vi "HFRR ADV v03.vi"() -> ()   [LabVIEW 2025] (continued)
            n1403 = Delete From Array(array=w1051, index=0) -> (array with subset deleted=w926:dbl[])  [unwired: 1 in, 1 out]
            n1404 = Delete From Array(array=w1031, index=0) -> (array with subset deleted=w1011:dbl[])  [unwired: 1 in, 1 out]
            n1405 = Delete From Array(array=w1001, index=0) -> (array with subset deleted=w928:dbl[])  [unwired: 1 in, 1 out]
            n1406 = Delete From Array(array=w1039, index=0) -> (array with subset deleted=w1012:dbl[])  [unwired: 1 in, 1 out]
            n1407 = Delete From Array(array=w1049, index=0) -> (array with subset deleted=w1010:dbl[])  [unwired: 1 in, 1 out]
            n1408 = Delete From Array(array=w1058, index=0) -> (array with subset deleted=w1013:dbl[])  [unwired: 1 in, 1 out]
            n1409 = Bundle "Bundle"(w922, w1011) -> (w1076:cluster{dbl[], dbl[]})  [unwired: 1 in]
            n1410 = Bundle "Bundle"(w926, w1010) -> (w1078:cluster{dbl[], dbl[]})  [unwired: 1 in]
            n1411 = Bundle "Bundle"(w924, w1012) -> (w1077:cluster{dbl[], dbl[]})  [unwired: 1 in]
            n1412 = Bundle "Bundle"(w928, w1013) -> (w947:cluster{dbl[], dbl[]})  [unwired: 1 in]
            n1413 = Build Array "Build Array"(w947, w1078, w1077, w1076) -> (→"Coefficient Of Friction":cluster{dbl[], dbl[]}[])
            n1414 = Delete From Array(array=w1046, index=0) -> (array with subset deleted=w1047:dbl[])  [unwired: 1 in, 1 out]
            n1415 = Delete From Array(array=w1028, index=0) -> (array with subset deleted=w1029:dbl[])  [unwired: 1 in, 1 out]
            n1416 = Delete From Array(array=w1037, index=0) -> (array with subset deleted=w1038:dbl[])  [unwired: 1 in, 1 out]
            n1417 = Delete From Array(array=w1055, index=0) -> (array with subset deleted=w1056:dbl[])  [unwired: 1 in, 1 out]
            n1418 = Delete From Array(array=w1026, index=0) -> (array with subset deleted=w956:dbl[])  [unwired: 1 in, 1 out]
            n1419 = Delete From Array(array=w1035, index=0) -> (array with subset deleted=w957:dbl[])  [unwired: 1 in, 1 out]
            n1420 = Delete From Array(array=w1053, index=0) -> (array with subset deleted=w959:dbl[])  [unwired: 1 in, 1 out]
            n1421 = Delete From Array(array=w1044, index=0) -> (array with subset deleted=w958:dbl[])  [unwired: 1 in, 1 out]
            n1422 = Bundle "Bundle"(w922, w956) -> (w1068:cluster{dbl[], dbl[]})  [unwired: 1 in]
            n1423 = Bundle "Bundle"(w926, w958) -> (w1069:cluster{dbl[], dbl[]})  [unwired: 1 in]
            n1424 = Bundle "Bundle"(w924, w957) -> (w1067:cluster{dbl[], dbl[]})  [unwired: 1 in]
            n1425 = Bundle "Bundle"(w928, w959) -> (w946:cluster{dbl[], dbl[]})  [unwired: 1 in]
            n1426 = Delete From Array(array=w1019, index=0) -> (array with subset deleted=w1007:dbl[])  [unwired: 1 in, 1 out]
            n1427 = Build Array "Build Array"(w946, w1069, w1067, w1068) -> (→"Air Temperature":cluster{dbl[], dbl[]}[])
            n1428 = Delete From Array(array=w1024, index=0) -> (array with subset deleted=w1009:dbl[])  [unwired: 1 in, 1 out]
            "array w/ subset deleted" <- w1009
            n1429 = Delete From Array(array=w1022, index=0) -> (array with subset deleted=w1008:dbl[])  [unwired: 1 in, 1 out]
            n1430 = Delete From Array(array=w999, index=0) -> (array with subset deleted=w955:dbl[])  [unwired: 1 in, 1 out]
            n1431 = Bundle "Bundle"(w922, w1029) -> (w1061:cluster{dbl[], dbl[]})  [unwired: 1 in]
            n1432 = Bundle "Bundle"(w926, w1047) -> (w1060:cluster{dbl[], dbl[]})  [unwired: 1 in]
            n1433 = Bundle "Bundle"(w924, w1038) -> (w1062:cluster{dbl[], dbl[]})  [unwired: 1 in]
            n1434 = Bundle "Bundle"(w928, w1056) -> (w920:cluster{dbl[], dbl[]})  [unwired: 1 in]
            n1435 = Build Array "Build Array"(w920, w1060, w1062, w1061) -> (→"XY Graph 13":cluster{dbl[], dbl[]}[])
            n1436 = Delete From Array(array=w1018, index=0) -> (array with subset deleted=w1006:dbl[])  [unwired: 1 in, 1 out]
            n1437 = Delete From Array(array=w993, index=0) -> (array with subset deleted=w952:dbl[])  [unwired: 1 in, 1 out]
            n1438 = Delete From Array(array=w997, index=0) -> (array with subset deleted=w954:dbl[])  [unwired: 1 in, 1 out]
            n1439 = Delete From Array(array=w995, index=0) -> (array with subset deleted=w953:dbl[])  [unwired: 1 in, 1 out]
            n1440 = call-poly <vilib>:"Mean.vi"("X"=w1011) -> ("mean"=→"КОФ4":dbl)  [unwired: 1 out]
            n1441 = call-poly <vilib>:"Mean.vi"("X"=w1013) -> ("mean"=→"КОФ1":dbl)  [unwired: 1 out]
            n1442 = call-poly <vilib>:"Mean.vi"("X"=w1012) -> ("mean"=→"КОФ3":dbl)  [unwired: 1 out]
            n1443 = Bundle "Bundle"(w928, w1009) -> (w942:cluster{dbl[], dbl[]})  [unwired: 1 in]
            n1444 = Bundle "Bundle"(w922, w1006) -> (w1014:cluster{dbl[], dbl[]})  [unwired: 1 in]
            n1445 = Bundle "Bundle"(w926, w1008) -> (w1016:cluster{dbl[], dbl[]})  [unwired: 1 in]
            n1446 = Bundle "Bundle"(w924, w1007) -> (w1015:cluster{dbl[], dbl[]})  [unwired: 1 in]
            n1447 = call-poly <vilib>:"Mean.vi"("X"=w1010) -> ("mean"=→"КОФ2":dbl)  [unwired: 1 out]
            n1448 = Build Array "Build Array"(w942, w1016, w1015, w1014) -> (→"Sample Temperature":cluster{dbl[], dbl[]}[])
            n1449 = Bundle "Bundle"(w928, w955) -> (w919:cluster{dbl[], dbl[]})  [unwired: 1 in]
            n1450 = Bundle "Bundle"(w922, w952) -> (w990:cluster{dbl[], dbl[]})  [unwired: 1 in]
            n1451 = Bundle "Bundle"(w926, w954) -> (w992:cluster{dbl[], dbl[]})  [unwired: 1 in]
            n1452 = Bundle "Bundle"(w924, w953) -> (w991:cluster{dbl[], dbl[]})  [unwired: 1 in]
            n1453 = Delete From Array(array=w978, index=0) -> (array with subset deleted=w950:dbl[])  [unwired: 1 in, 1 out]
            n1454 = Delete From Array(array=w976, index=0) -> (array with subset deleted=w949:dbl[])  [unwired: 1 in, 1 out]
            n1455 = call-poly <vilib>:"Mean.vi"("X"=w1008) -> ("mean"=→"CP2":dbl)  [unwired: 1 out]
            n1456 = call-poly <vilib>:"Mean.vi"("X"=w1006) -> ("mean"=→"CP4":dbl)  [unwired: 1 out]
            n1457 = Build Array "Build Array"(w919, w992, w991, w990) -> (→"Humidity":cluster{dbl[], dbl[]}[])
            n1458 = call-poly <vilib>:"Mean.vi"("X"=w1007) -> ("mean"=→"CP3":dbl)  [unwired: 1 out]
            n1459 = call-poly <vilib>:"Mean.vi"("X"=w1009) -> ("mean"=→"CP1":dbl)  [unwired: 1 out]
            n1460 = Delete From Array(array=w980, index=0) -> (array with subset deleted=w951:dbl[])  [unwired: 1 in, 1 out]
            n1461 = Bundle "Bundle"(w959, w955) -> (w961:cluster{dbl[], dbl[]})  [unwired: 1 in]
            n1462 = Bundle "Bundle"(w956, w952) -> (w964:cluster{dbl[], dbl[]})  [unwired: 1 in]
            n1463 = Bundle "Bundle"(w958, w954) -> (w962:cluster{dbl[], dbl[]})  [unwired: 1 in]
            n1464 = Bundle "Bundle"(w957, w953) -> (w963:cluster{dbl[], dbl[]})  [unwired: 1 in]
            n1465 = Delete From Array(array=w974, index=0) -> (array with subset deleted=w948:dbl[])  [unwired: 1 in, 1 out]
            n1466 = Build Array "Build Array"(w961, w962, w963, w964) -> (→"Air Temp vs Rh":cluster{dbl[], dbl[]}[])
            n1467 = Build Array "Build Array"(w919, w942) -> (w945:cluster{dbl[], dbl[]}[])
            "XY Graph 17" <- w945
            n1468 = local write "XY Graph 16"(w945) -> ()
            n1469 = Bundle "Bundle"(w926, w950) -> (w972:cluster{dbl[], dbl[]})  [unwired: 1 in]
            n1470 = Bundle "Bundle"(w924, w949) -> (w971:cluster{dbl[], dbl[]})  [unwired: 1 in]
            n1471 = Bundle "Bundle"(w922, w948) -> (w970:cluster{dbl[], dbl[]})  [unwired: 1 in]
            n1472 = Bundle "Bundle"(w928, w951) -> (w973:cluster{dbl[], dbl[]})  [unwired: 1 in]
            n1473 = Delete From Array(array=w940, index=0) -> (array with subset deleted=w927:dbl[])  [unwired: 1 in, 1 out]
            n1474 = Delete From Array(array=w936, index=0) -> (array with subset deleted=w925:dbl[])  [unwired: 1 in, 1 out]
            n1475 = Build Array "Build Array"(w973, w972, w971, w970) -> (→"Stroke":cluster{dbl[], dbl[]}[])
            n1476 = Delete From Array(array=w934, index=0) -> (array with subset deleted=w921:dbl[])  [unwired: 1 in, 1 out]
            n1477 = Delete From Array(array=w935, index=0) -> (array with subset deleted=w923:dbl[])  [unwired: 1 in, 1 out]
            n1478 = Bundle "Bundle"(w928, w927) -> (w933:cluster{dbl[], dbl[]})  [unwired: 1 in]
            n1479 = Bundle "Bundle"(w926, w925) -> (w932:cluster{dbl[], dbl[]})  [unwired: 1 in]
            n1480 = call-poly <vilib>:"Mean.vi"("X"=w951) -> ("mean"=→"КОФ2 2":dbl)  [unwired: 1 out]
            n1481 = Bundle "Bundle"(w922, w921) -> (w930:cluster{dbl[], dbl[]})  [unwired: 1 in]
            n1482 = Bundle "Bundle"(w924, w923) -> (w931:cluster{dbl[], dbl[]})  [unwired: 1 in]
            n1483 = call-poly <vilib>:"Mean.vi"("X"=w950) -> ("mean"=→"КОФ2 3":dbl)  [unwired: 1 out]
            n1484 = call-poly <vilib>:"Mean.vi"("X"=w948) -> ("mean"=→"КОФ2 5":dbl)  [unwired: 1 out]
            n1485 = call-poly <vilib>:"Mean.vi"("X"=w949) -> ("mean"=→"КОФ2 4":dbl)  [unwired: 1 out]
            n1486 = Build Array "Build Array"(w933, w932, w931, w930) -> (→"Frequency":cluster{dbl[], dbl[]}[])
          }
          frame #2 {
          }
          frame #3 {
            n1487 = local read "String Control 4"() -> (w1244:string)
            n1488 = local read "String Control 6"() -> (w1243:string)
            n1489 = local read "String Control 8"() -> (w1242:string)
            n1490 = local read "String Control 2"() -> (w1245:string)
            n1491 = property on="OPEN" class="Bool (strict)"("Visible"=TRUE) -> ()  [unwired: 2 in, 2 out]
            n1492 = Match Pattern(string=w1243, regular expression="Frequency :- ") -> (after substring=w1268:string)  [unwired: 1 in, 3 out]
            n1493 = Match Pattern(string=w1245, regular expression="Frequency :- ") -> (after substring=w1278:string)  [unwired: 1 in, 3 out]
            n1494 = Match Pattern(string=w1244, regular expression="Frequency :- ") -> (after substring=w1273:string)  [unwired: 1 in, 3 out]
            n1495 = Match Pattern(string=w1242, regular expression="Frequency :- ") -> (after substring=w1263:string)  [unwired: 1 in, 3 out]
            n1496 = String Subset(string=w1268, length (rest)=9 ("length (rest)")) -> (substring=w1270:string)  [unwired: 1 in]
            n1497 = String Subset(string=w1278, length (rest)=9 ("length (rest)")) -> (substring=w1280:string)  [unwired: 1 in]
            n1498 = String Subset(string=w1273, length (rest)=9 ("length (rest)")) -> (substring=w1275:string)  [unwired: 1 in]
            n1499 = String Subset(string=w1263, length (rest)=9 ("length (rest)")) -> (substring=w1265:string)  [unwired: 1 in]
            n1500 = Fract/Exp String To Number(string=w1270) -> (number=w1271:dbl)  [unwired: 3 in, 1 out]
            n1501 = Fract/Exp String To Number(string=w1280) -> (number=w1281:dbl)  [unwired: 3 in, 1 out]
            n1502 = Fract/Exp String To Number(string=w1275) -> (number=w1276:dbl)  [unwired: 3 in, 1 out]
            n1503 = Fract/Exp String To Number(string=w1265) -> (number=w1266:dbl)  [unwired: 3 in, 1 out]
            n1504 = local write "freq3"(w1271) -> ()
            n1505 = local write "freq2"(w1276) -> ()
            n1506 = local write "freq1"(w1281) -> ()
            n1507 = local write "freq 4"(w1266) -> ()
            n1508 = local write "Numeric 13"(0 ("Numeric 13")) -> ()
            n1509 = local write "Numeric 11"(0 ("Numeric 11")) -> ()
            n1510 = local write "Numeric 8"(0 ("Numeric 8")) -> ()
            n1511 = local write "Numeric 12"(0 ("Numeric 12")) -> ()
            n1512 = Match Pattern(string=w1243, regular expression="Samples / cycle :- ") -> (after substring=w1251:string)  [unwired: 1 in, 3 out]
            n1513 = Match Pattern(string=w1245, regular expression="Samples / cycle :- ") -> (after substring=w1259:string)  [unwired: 1 in, 3 out]
            n1514 = Match Pattern(string=w1244, regular expression="Samples / cycle :- ") -> (after substring=w1255:string)  [unwired: 1 in, 3 out]
            n1515 = Match Pattern(string=w1242, regular expression="Samples / cycle :- ") -> (after substring=w1247:string)  [unwired: 1 in, 3 out]
            n1516 = String Subset(string=w1251, length (rest)=6 ("length (rest)")) -> (substring=w1253:string)  [unwired: 1 in]
            n1517 = String Subset(string=w1259, length (rest)=6 ("length (rest)")) -> (substring=w1261:string)  [unwired: 1 in]
            n1518 = String Subset(string=w1255, length (rest)=6 ("length (rest)")) -> (substring=w1257:string)  [unwired: 1 in]
            n1519 = String Subset(string=w1247, length (rest)=6 ("length (rest)")) -> (substring=w1249:string)  [unwired: 1 in]
            n1520 = Fract/Exp String To Number(string=w1253) -> (number=w1239:dbl)  [unwired: 3 in, 1 out]
            n1521 = Fract/Exp String To Number(string=w1261) -> (number=w1241:dbl)  [unwired: 3 in, 1 out]
            n1522 = Fract/Exp String To Number(string=w1257) -> (number=w1240:dbl)  [unwired: 3 in, 1 out]
            n1523 = Fract/Exp String To Number(string=w1249) -> (number=w1238:dbl)  [unwired: 3 in, 1 out]
            n1524 = local write "sample2"(w1240) -> ()
            n1525 = local write "sample3"(w1239) -> ()
            n1526 = local write "sample1"(w1241) -> ()
            n1527 = local write "sample4"(w1238) -> ()
          }
        }
      }
    }
    n1528 = Wait (ms)(milliseconds to wait=u32 50) -> ()  [unwired: 1 out]
    n1529 = property on="STOP 3" class="Bool (strict)"() -> ("Visible"=w852:bool)  [unwired: 2 in, 2 out]
    n1530 = case shown="True" w852 {
      frame False {
      }
      frame True {
        n1531 = case shown="True" "Save Results" {
          frame False {
          }
          frame True {
            w1765 = "\r"
            n1532 = local read "Temperature before test"() -> (w1803:dbl)
            n1533 = local read "Temperature after test"() -> (w1805:dbl)
            n1534 = local read "Humidity before test"() -> (w1802:dbl)
            n1535 = local read "Humidity after test"() -> (w1804:dbl)
            n1536 = local read "MWSD"() -> (w1806:dbl)
            n1537 = local read "WS1.4"() -> (w1809:dbl)
            n1538 = local read "AVP"() -> (w1807:dbl)
            n1539 = local read "HCF"() -> (w1808:dbl)
            n1540 = local write "Save Results"(FALSE ("OK Button 5")) -> ()
            n1541 = Number To Fractional String(number=w1805, width (-)=i16 6, precision (6)=i16 1) -> (F-format string=w1783:string)  [unwired: 1 in]
            n1542 = Number To Fractional String(number=w1806, width (-)=i16 6, precision (6)=i16 1) -> (F-format string=w1780:string)  [unwired: 1 in]
            n1543 = Number To Fractional String(number=w1807, width (-)=i16 6, precision (6)=i16 3) -> (F-format string=w1776:string)  [unwired: 1 in]
            n1544 = Number To Fractional String(number=w1804, width (-)=i16 6, precision (6)=i16 1) -> (F-format string=w1787:string)  [unwired: 1 in]
            n1545 = Number To Fractional String(number=w1808, width (-)=i16 6, precision (6)=i16 2) -> (F-format string=w1774:string)  [unwired: 1 in]
            n1546 = Number To Fractional String(number=w1809, width (-)=i16 6, precision (6)=i16 1) -> (F-format string=w1769:string)  [unwired: 1 in]
            n1547 = Number To Fractional String(number=w1803, width (-)=i16 6, precision (6)=i16 1) -> (F-format string=w1791:string)  [unwired: 1 in]
            n1548 = Number To Fractional String(number=w1802, width (-)=i16 6, precision (6)=i16 1) -> (F-format string=w1794:string)  [unwired: 1 in]
            n1549 = local read "String"() -> (w1798:string)
            n1550 = local read "FILE"() -> (w1801:string)
            n1551 = Concatenate Strings(w1798, w1801) -> (w1820:string)
            n1552 = Concatenate Strings(w1820, ".dwm" ("Substring")) -> (w1818:string)
            n1553 = Concatenate Strings(w1774, ")" ("string")) -> (w1772:string)
            n1554 = Concatenate Strings("(" ("string"), w1769, ")Microns" ("string")) -> (w1768:string)
            n1555 = Concatenate Strings("(" ("string"), w1794, " ) % RH," ("string")) -> (w1795:string)
            n1556 = Concatenate Strings("(" ("string"), w1776, ")  kPa," ("string")) -> (w1766:string)
            n1557 = String To Path(string=w1818) -> (path=w1817:path)
            n1558 = Concatenate Strings("(" ("string"), w1791, ")  Deg C ," ("string")) -> (w1790:string)
            n1559 = Concatenate Strings("(" ("string"), w1787, " ) % RH," ("string")) -> (w1786:string)
            n1560 = Concatenate Strings("(" ("string"), w1783, ")  Deg C ," ("string")) -> (w1782:string)
            n1561 = Concatenate Strings("(" ("string"), w1780, ")  Microns," ("string")) -> (w1779:string)
            n1562 = local read "REMARKS"() -> (w1800:string)
            "REMARKS 2" <- w1800
            n1563 = Concatenate Strings(w1800, w1765, " Humidity before test= " ("Substring"), w1795, w1765, " Temperature before test = " ("Substring"), w1790, w1765, " Humidity after test= " ("Substring"), w1786, w1765, "Temperature after test = " ("Substring"), w1782, w1765, "MSD = " ("Substring"), w1779, w1765, "  AVP = " ("Substring"), w1766, w1765, "  HCF                     =( " ("Substring"), w1772, w1765, " WS1.4                  = " ("Substring"), w1768, w1765) -> (w1764:string)
            "data" <- w1764
            n1564 = call <vilib>:"Write Characters To File.vi"("append to file? (new file:F)"=FALSE, "character string"=w1764, "file path (dialog if empty)"=w1817) -> ()  [unwired: 2 in, 1 out]
            n1565 = Match Pattern(string=w1764, regular expression="!") -> (after substring=→"export":string)  [unwired: 1 in, 3 out]
          }
        }
        n1566 = local read "Temperature before test"() -> (w1733:dbl)
        n1567 = local read "Humidity before test"() -> (w1735:dbl)
        n1568 = local read "Temperature after test"() -> (w1749:dbl)
        n1569 = Add(x=231.864, y=w1733) -> (x+y=w1730:dbl)
        n1570 = Add(x=231.864, y=w1749) -> (x+y=w1746:dbl)
        n1571 = local read "Humidity after test"() -> (w1751:dbl)
        n1572 = Divide(x=1705.984, y=w1730) -> (x/y=w1731:dbl)
        n1573 = Divide(x=1705.984, y=w1746) -> (x/y=w1747:dbl)
        n1574 = Subtract(x=8.017352 ("y"), y=w1731) -> (x-y=w1760:dbl)
        n1575 = expression code="10**y"(w1760) -> (w1737:dbl)
        n1576 = Subtract(x=8.017352 ("y"), y=w1747) -> (x-y=w1754:dbl)
        n1577 = expression code="10**y"(w1754) -> (w1753:dbl)
        n1578 = Multiply(x=w1735, y=w1737) -> (x*y=w1736:dbl)
        n1579 = Multiply(x=w1751, y=w1753) -> (x*y=w1752:dbl)
        n1580 = Divide(x=w1736, y=750.0) -> (x/y=w1755:dbl)
        n1581 = Divide(x=w1752, y=750.0) -> (x/y=w1756:dbl)
        n1582 = Add(x=w1755, y=w1756) -> (x+y=w1757:dbl)
        n1583 = Divide(x=w1757, y=2.0) -> (x/y=w1759:dbl)
        n1584 = local write "AVP"(w1759) -> ()
        n1585 = local read "HCF"() -> (w1742:dbl)
        n1586 = Subtract(x=1.4, y=w1759) -> (x-y=w1740:dbl)
        n1587 = local read "MWSD"() -> (w1738:dbl)
        n1588 = Multiply(x=w1740, y=w1742) -> (x*y=w1741:dbl)
        n1589 = Add(x=w1741, y=w1738) -> (x+y=→"WS1.4":dbl)
      }
    }
    n1590 = case shown="True" "Prog Uno" {
      frame False {
      }
      frame True {
        n1591 = stacked-sequence {
          frame #0 {
            n1592 = Delete(path (use dialog)=path "C:/LAB-IQ-NXT/UNOCOMPILE.bat" ("working directory")) -> ()  [unwired: 4 in, 3 out]
          }
          frame #1 {
            n1593 = local read "Com Port 1"() -> (w1332:refnum<visa-resource-name>)
            n1594 = Concatenate Strings("cmd.exe /c \"mode " ("command line"), w1332, ":1200,n,8,1\"\n" ("command line")) -> (w1337:string)
            n1595 = Concatenate Strings(w1337, "CD\\\nCD WinDucom\navrdude -C avrdude.conf -v -patmega328p -carduino -P" ("command line"), w1332, " -b115200 -D -Uflash:w:UNO_V20.hex:i\n" ("command line"), "\r") -> (w1339:string)
            "STR" <- w1339
            n1596 = call <vilib>:"Write Characters To File.vi"("append to file? (new file:F)"=FALSE, "character string"=w1339, "file path (dialog if empty)"=path "C:/LAB-IQ-NXT/UNOCOMPILE.bat" ("working directory")) -> ()  [unwired: 2 in, 1 out]
          }
          frame #2 {
            n1597 = case shown="True" "Case Constant\n(See Context Help) 10" {
              frame False {
              }
              frame True {
                w1345 = "cmd.exe  /c \"C:\\LAB-IQ-NXT\\UNOCOMPILE.bat\"" ("string")
                n1598 = call <vilib>:"System Exec.vi"("expected output size  (4096)"=u32 65535, "run minimized? (F)"=FALSE, "wait until completion? (T)"=TRUE ("run minimized? (F)"), "working directory"=path "C:/LAB-IQ-NXT", "standard input"=w1345, "command line"=w1345) -> ("error out"=w1344:errorcluster, "standard output"=→"String 42":string)  [unwired: 2 in, 2 out]
                "error out 3" <- w1344
                n1599 = flat-sequence {
                  tunnel: w1344 -> [_]
                  frame #0 {
                  }
                }
              }
            }
            n1600 = local write "Prog Uno"(FALSE ("run minimized? (F)")) -> ()
          }
        }
      }
    }
    n1601 = case shown="True" "Prog Due" {
      frame False {
      }
      frame True {
        n1602 = stacked-sequence {
          frame #0 {
            n1603 = Delete(path (use dialog)=path "C:/LAB-IQ-NXT/DUECOMPILE.bat" ("working directory")) -> ()  [unwired: 4 in, 3 out]
          }
          frame #1 {
            n1604 = case shown="True" "Case Constant\n(See Context Help) 11" {
              frame False {
              }
              frame True {
                n1605 = local read "visa due"() -> (w1313:string)
                n1606 = Concatenate Strings("cmd.exe /c \"mode " ("command line"), w1313, ":1200,n,8,1\"\n" ("command line")) -> (w1318:string)
                n1607 = Concatenate Strings(w1318, "CD\\\nCD WinDucom\nTIMEOUT 1\n bossac.exe -i -d --port=" ("command line"), w1313, " -U false -e -w -v -b DUE.bin -R\n" ("command line"), "\r") -> (w1320:string)
                "concatenated string 2" <- w1320
                n1608 = call <vilib>:"Write Characters To File.vi"("append to file? (new file:F)"=FALSE, "character string"=w1320, "file path (dialog if empty)"=path "C:/LAB-IQ-NXT/DUECOMPILE.bat" ("working directory")) -> ()  [unwired: 2 in, 1 out]
              }
            }
          }
          frame #2 {
            # "C:\\LAB-IQ-NXT\\DUECOMPILE.bat"
            n1609 = case shown="True" "Case Constant\n(See Context Help) 12" {
              frame False {
              }
              frame True {
                w1326 = "cmd.exe  /c \"C:\\LAB-IQ-NXT\\DUECOMPILE.bat\"" ("string")
                n1610 = call <vilib>:"System Exec.vi"("expected output size  (4096)"=u32 65535, "run minimized? (F)"=FALSE, "wait until completion? (T)"=TRUE ("run minimized? (F)"), "working directory"=path "C:/LAB-IQ-NXT", "standard input"=w1326, "command line"=w1326) -> ("error out"=w1325:errorcluster, "standard output"=→"String 44":string)  [unwired: 2 in, 2 out]
                "error out 4" <- w1325
                n1611 = flat-sequence {
                  tunnel: w1325 -> [_]
                  frame #0 {
                  }
                }
              }
            }
            n1612 = local write "Prog Due"(FALSE ("Prog Due")) -> ()
          }
        }
      }
    }
    n1613 = flat-sequence {
      frame #0 {
        n1614 = local read "x = y?"() -> (w1355:bool)
        n1615 = And(x="EDIT", y=w1355) -> (x .and. y?=w1353:bool)
        n1616 = case shown="True" "SAVE" {
          frame False {
          }
          frame True {
            n1617 = stacked-sequence {
              seq-local: [w1556 _ _] -> [_ w1710 _]
              frame #0 {
                (unwired) i16 5 ("precision (6)")
                # "[CH1]    - FF\n[CH2]   - TEMPERATURE\n[CH3]    - Humidity\n[CH4]    - AIR TEMP\n[CH5]\\- Visa Uno\n[CH6] \\- Visa Due\n[CH7]  \\- file path\n[CH8]   - Displacement Gain\n[CHA]   - Stroke Gain\n[CHB]   - Stroke PID Gain\n[CHC]   -Language Selection\n[CHD]   -Power +\n[CHE]   -Power_\n[CHF]   -Heater\n[CHG]   -Humidity Wet\n[CHH]   -Humidity Dry\n[CHI]   -Integral Time"
                n1618 = local read "Com Port 1"() -> (w1547:refnum<visa-resource-name>)
                n1619 = local read "AIR TEMPERATURE :"() -> (w1543:dbl)
                n1620 = local read "DISPLACEMENT :"() -> (w1541:dbl)
                n1621 = local read "HUMIDITY:"() -> (w1542:dbl)
                n1622 = local read "Com Port 2"() -> (w1546:refnum<visa-resource-name>)
                n1623 = local read "TEMPERATURE :"() -> (w1544:dbl)
                n1624 = local read "Stroke PID Gains"() -> (w1607:T5)
                n1625 = local read "FRIC. FORCE :"() -> (w1545:dbl)
                n1626 = local read "STROKE GAIN :"() -> (w1540:dbl)
                n1627 = Unbundle By Name(w1607) -> ("Proportional Gain (Kc)"=w1606:dbl, "Integral Time (Ti, min)"=w1548:dbl)
                n1628 = local read "CH-HUMIDITY DRY"() -> (w1559:u16)
                n1629 = Path To String(path="File Path") -> (string=w1629:string)
                n1630 = local read "Language Selection"() -> (w1604:enum16{"English", "Russian"})
                n1631 = local read "CH-POWER +"() -> (w1571:u16)
                n1632 = local read "CH-HUMIDITY WET"() -> (w1562:u16)
                n1633 = Number To Fractional String(number=w1542, width (-)=i16 10 ("precision (6)"), precision (6)=i16 5) -> (F-format string=w1654:string)  [unwired: 1 in]
                n1634 = Concatenate Strings(w1629, "\\" ("string")) -> (w1628:string)
                n1635 = local read "CH-POWER -"() -> (w1568:u16)
                n1636 = Number To Fractional String(number=w1544, width (-)=i16 10 ("precision (6)"), precision (6)=i16 5) -> (F-format string=w1660:string)  [unwired: 1 in]
                n1637 = Number To Fractional String(number=w1543, width (-)=i16 10 ("precision (6)"), precision (6)=i16 5) -> (F-format string=w1648:string)  [unwired: 1 in]
                n1638 = Number To Fractional String(number=w1541, width (-)=i16 10 ("precision (6)"), precision (6)=i16 5) -> (F-format string=w1621:string)  [unwired: 1 in]
                n1639 = local read "CH-HEATER"() -> (w1565:u16)
                n1640 = Number To Fractional String(number=w1540, width (-)=i16 10 ("precision (6)"), precision (6)=i16 5) -> (F-format string=w1620:string)  [unwired: 1 in]
                n1641 = Number To Fractional String(number=w1545, width (-)=i16 10 ("precision (6)"), precision (6)=i16 5) -> (F-format string=w1661:string)  [unwired: 1 in]
                n1642 = Number To Fractional String(number=w1606, width (-)=i16 10 ("precision (6)"), precision (6)=i16 5) -> (F-format string=w1608:string)  [unwired: 1 in]
                n1643 = Number To Fractional String(number=w1604, width (-)=i16 10 ("precision (6)"), precision (6)=i16 5) -> (F-format string=w1600:string)  [unwired: 1 in]
                n1644 = Number To Fractional String(number=w1571, width (-)=i16 10 ("precision (6)"), precision (6)=i16 5) -> (F-format string=w1594:string)  [unwired: 1 in]
                n1645 = Number To Fractional String(number=w1568, width (-)=i16 10 ("precision (6)"), precision (6)=i16 5) -> (F-format string=w1591:string)  [unwired: 1 in]
                n1646 = Number To Fractional String(number=w1565, width (-)=i16 10 ("precision (6)"), precision (6)=i16 5) -> (F-format string=w1586:string)  [unwired: 1 in]
                n1647 = Number To Fractional String(number=w1562, width (-)=i16 10 ("precision (6)"), precision (6)=i16 5) -> (F-format string=w1583:string)  [unwired: 1 in]
                n1648 = Number To Fractional String(number=w1559, width (-)=i16 10 ("precision (6)"), precision (6)=i16 5) -> (F-format string=w1578:string)  [unwired: 1 in]
                n1649 = Concatenate Strings("[CH1]" ("string"), w1661, " - FF" ("string"), "\r") -> (w1659:string)
                n1650 = Concatenate Strings("[CH3]" ("string"), w1654, " - Humidity" ("string"), "\r") -> (w1651:string)
                n1651 = Concatenate Strings("[CH7]" ("string"), w1628, "- file path" ("string"), "\r") -> (w1631:string)
                n1652 = Number To Fractional String(number=w1548, width (-)=i16 10 ("precision (6)"), precision (6)=i16 5) -> (F-format string=w1552:string)  [unwired: 1 in]
                n1653 = Concatenate Strings("[CH6]" ("string"), w1546, "- Visa Due" ("string"), "\r") -> (w1632:string)
                n1654 = Concatenate Strings("[CH8]" ("string"), w1621, "- Displacement Gain" ("string"), "\r") -> (w1624:string)
                n1655 = Concatenate Strings("[CHA]" ("string"), w1620, "- Stroke Gain" ("string"), "\r") -> (w1614:string)
                n1656 = Concatenate Strings("[CH5]" ("string"), w1547, "- Visa Uno" ("string"), "\r") -> (w1637:string)
                n1657 = Concatenate Strings("[CH4]" ("string"), w1648, " - AIR TEMP" ("string"), "\r") -> (w1644:string)
                n1658 = Concatenate Strings("[CH2]" ("string"), w1660, " - TEMPERATURE" ("string"), "\r") -> (w1658:string)
                n1659 = Concatenate Strings("[CHC]" ("string"), w1600, "-Language Selection" ("string"), "\r") -> (w1597:string)
                n1660 = Concatenate Strings("[CHD]" ("string"), w1594, "-Power +" ("string"), "\r") -> (w1576:string)
                n1661 = Concatenate Strings("[CHE]" ("string"), w1591, "-Power_" ("string"), "\r") -> (w1575:string)
                n1662 = Concatenate Strings("[CHF]" ("string"), w1586, "-Heater" ("string"), "\r") -> (w1574:string)
                n1663 = Concatenate Strings("[CHB]" ("string"), w1608, "- Stroke PID Gain" ("string"), "\r") -> (w1605:string)
                n1664 = Concatenate Strings("[CHG]" ("string"), w1583, "-Humidity Wet" ("string"), "\r") -> (w1573:string)
                n1665 = Concatenate Strings("[CHH]" ("string"), w1578, "-Humidity Dry" ("string"), "\r") -> (w1572:string)
                n1666 = Concatenate Strings("[CHI]" ("string"), w1552, "-Integral Time " ("string"), "\r") -> (w1549:string)
                n1667 = Concatenate Strings(w1659, w1658, w1651, w1644, w1637, w1632, w1631, w1624, w1614, w1605, w1597, w1576, w1575, w1574, w1573, w1572, w1549) -> (w1556:string)
                "gain" <- w1556
              }
              frame #1 {
                n1668 = local read "AIR TEMP INTERCEPT:"() -> (w1673:dbl)
                n1669 = local read "TEMP INTERCEPT:"() -> (w1672:dbl)
                n1670 = local read "Com Port 3"() -> (w1682:refnum<visa-resource-name>)
                n1671 = local read "LvdtOff"() -> (w1675:dbl)
                n1672 = Number To Fractional String(number=w1672, width (-)=i16 10 ("precision (6)"), precision (6)=i16 5) -> (F-format string=w1698:string)  [unwired: 1 in]
                n1673 = Number To Fractional String(number=w1673, width (-)=i16 10 ("precision (6)"), precision (6)=i16 5) -> (F-format string=w1705:string)  [unwired: 1 in]
                n1674 = Number To Fractional String(number=w1675, width (-)=i16 10 ("precision (6)"), precision (6)=i16 5) -> (F-format string=w1679:string)  [unwired: 1 in]
                n1675 = Concatenate Strings("[CHK]" ("string"), w1698, "-TEMP INTERCEPT" ("string"), "\r") -> (w1694:string)
                n1676 = Concatenate Strings("[CHJ]" ("string"), w1705, "-AIR TEMP INTERCEPT" ("string"), "\r") -> (w1695:string)
                n1677 = Concatenate Strings("[SNO]" ("string"), "S.NO", "-" ("string"), "\r") -> (w1690:string)
                n1678 = Concatenate Strings("[CHL]" ("string"), w1682, "- Visa humid" ("string"), "\r") -> (w1685:string)
                n1679 = Concatenate Strings("[CHI]" ("string"), w1679, "-LVDT Position Offset" ("string"), "\r") -> (w1674:string)
                n1680 = Concatenate Strings(w1710, w1695, w1694, w1690, w1685, w1674) -> (w1709:string)
                n1681 = String To Path(string="C:\\LAB-IQ-NXT\\calibrate WO 2464.dcf") -> (path=w1683:path)
                n1682 = call <vilib>:"Write Characters To File.vi"("append to file? (new file:F)"=FALSE, "character string"=w1709, "file path (dialog if empty)"=w1683) -> ()  [unwired: 2 in, 1 out]
              }
              frame #2 {
                n1683 = local write "Lan flag"(0.0 ("Lan flag")) -> ()
                n1684 = local write "Re-Initialise"(TRUE ("Re-Initialise")) -> ()
                n1685 = local write "conststatus"(0.0 ("rpm value : 2")) -> ()
                n1686 = local write "SAVE"(FALSE ("OK Button 14")) -> ()
              }
            }
          }
        }
        n1687 = case shown="False" w1353 {
          tunnel: [u8 2 ("Disabled") u8 0 ("Disabled")] -> w1352
          tunnel: [w1715 TRUE ("Visible")] -> w1351
          frame False {
            w1715 = FALSE ("Visible")
            n1688 = local write "EDIT 2"(w1715) -> ()
          }
          frame True {
          }
        }
        n1689 = property on="Tab Control" class="TabCtl (strict)"("Visible"=w1351) -> ()  [unwired: 2 in, 2 out]
        n1690 = property on="EDIT 2" class="Bool (strict)"("Visible"=w1351) -> ()  [unwired: 2 in, 2 out]
        n1691 = property on="TEMPERATURE :" class="DigNum (strict)"("Disabled"=w1352) -> ()  [unwired: 2 in, 2 out]
        n1692 = property on="SAVE" class="Bool (strict)"("Visible"=w1351) -> ()  [unwired: 2 in, 2 out]
        n1693 = property on="AIR TEMPERATURE :" class="DigNum (strict)"("Disabled"=w1352) -> ()  [unwired: 2 in, 2 out]
        n1694 = property on="SPEED OUT:" class="DigNum (strict)"("Disabled"=w1352) -> ()  [unwired: 2 in, 2 out]
        n1695 = property on="HUMIDITY:" class="DigNum (strict)"("Disabled"=w1352) -> ()  [unwired: 2 in, 2 out]
        n1696 = property on="FRIC. FORCE :" class="DigNum (strict)"("Disabled"=w1352) -> ()  [unwired: 2 in, 2 out]
        n1697 = property on="Tab Control 7" class="TabCtl (strict)"("Disabled"=w1352) -> ()  [unwired: 2 in, 2 out]
        n1698 = property on="Language Selection" class="Enum (strict)"("Visible"=w1351) -> ()  [unwired: 2 in, 2 out]
        n1699 = property on="File Path" class="Path"("Disabled"=w1352) -> ()  [unwired: 2 in, 2 out]
        n1700 = property on="TEMP INTERCEPT:" class="DigNum (strict)"("Disabled"=w1352) -> ()  [unwired: 2 in, 2 out]
        n1701 = property on="visa due" class="CmbBox"("Disabled"=w1352) -> ()  [unwired: 2 in, 2 out]
        n1702 = property on="AIR TEMP INTERCEPT:" class="DigNum (strict)"("Disabled"=w1352) -> ()  [unwired: 2 in, 2 out]
        n1703 = property on="CH-HUMIDITY DRY" class="DigNum (strict)"("Disabled"=w1352) -> ()  [unwired: 2 in, 2 out]
        n1704 = property on="CH-HUMIDITY WET" class="DigNum (strict)"("Disabled"=w1352) -> ()  [unwired: 2 in, 2 out]
        n1705 = property on="CH-POWER -" class="DigNum (strict)"("Disabled"=w1352) -> ()  [unwired: 2 in, 2 out]
        n1706 = property on="CH-HEATER" class="DigNum (strict)"("Disabled"=w1352) -> ()  [unwired: 2 in, 2 out]
        n1707 = property on="CH-POWER +" class="DigNum (strict)"("Disabled"=w1352) -> ()  [unwired: 2 in, 2 out]
        n1708 = property on="SrvM CP" class="Bool (strict)"("Disabled"=w1352) -> ()  [unwired: 2 in, 2 out]
        n1709 = property on="Stroke PID Gains" class="Clust (strict)"("Disabled"=w1352) -> ()  [unwired: 2 in, 2 out]
        n1710 = property on="STROKE GAIN :" class="DigNum (strict)"("Disabled"=w1352) -> ()  [unwired: 2 in, 2 out]
        n1711 = property on="LvdtOff" class="DigNum (strict)"("Disabled"=w1352) -> ()  [unwired: 2 in, 2 out]
        n1712 = property on="DISPLACEMENT :" class="DigNum (strict)"("Disabled"=w1352) -> ()  [unwired: 2 in, 2 out]
        n1713 = property on="Port 2 Error" class="Clust (strict)"("Visible"="EDIT") -> ()  [unwired: 2 in, 2 out]
        n1714 = property on="Port 1 Error" class="Clust (strict)"("Visible"="EDIT") -> ()  [unwired: 2 in, 2 out]
        n1715 = stacked-sequence {
          frame #0 {
            n1716 = local read "EDIT"() -> (w1403:bool)
            n1717 = case shown="True" w1403 {
              tunnel: [u8 2 ("Disabled") u8 0 ("Disabled")] -> _
              frame False {
                w1405 = FALSE
                n1718 = local write "Password"("") -> ()
                n1719 = property on="ENTER THE NEW PASSWORD" class="Str"("Visible"=w1405) -> ()  [unwired: 2 in, 2 out]
                n1720 = property on="ENTER CURRENT PASSWORD" class="Str"("Visible"=w1405) -> ()  [unwired: 2 in, 2 out]
                n1721 = property on="SrvM CP" class="Bool (strict)"("Visible"=w1405) -> ()  [unwired: 2 in, 2 out]
                n1722 = property on="Password" class="Str"("Visible"=w1405) -> ()  [unwired: 2 in, 2 out]
                n1723 = local write "x = y?"(w1405) -> ()
                n1724 = local write "SrvM CP"(w1405) -> ()
                n1725 = property on="message" class="Str"("Visible"=w1405) -> ()  [unwired: 2 in, 2 out]
              }
              frame True {
                w1408 = TRUE
                n1726 = property on="SrvM CP" class="Bool (strict)"("Visible"=w1408) -> ()  [unwired: 2 in, 2 out]
                n1727 = property on="Password" class="Str"("Visible"=w1408) -> ()  [unwired: 2 in, 2 out]
              }
            }
            "dipl pwd" <- "@143$\n" ("dipl pwd")
          }
          frame #1 {
            # "Gain password"
            n1728 = String To Byte Array(string="ENTER CURRENT PASSWORD") -> (unsigned byte array=w1413:u8[])
            n1729 = Search 1D Array(1D array=w1413, element=u8 10) -> (index of element=w1416:i32)  [unwired: 1 in]
            n1730 = Index Array(array=w1413, index=w1416) -> (element=w1412:u8)
            n1731 = Equal?(x=w1412, y=10) -> (x = y?=w1410:bool)
            n1732 = case shown="True" w1410 {
              frame False {
                n1733 = property on="ENTER THE NEW PASSWORD" class="Str"("Visible"=FALSE) -> ()  [unwired: 2 in, 2 out]
              }
              frame True {
                # "password"
                # "change password logic"
                n1734 = local read "dipl pwd"() -> (w1423:string)
                n1735 = local read "ENTER CURRENT PASSWORD"() -> (w1429:string)
                n1736 = String To Byte Array(string=w1429) -> (unsigned byte array=w1431:u8[])
                n1737 = Array Size(array=w1431) -> (size(s)=w1428:i32)
                n1738 = String To Byte Array(string=w1423) -> (unsigned byte array=w1424:u8[])
                n1739 = Array Size(array=w1424) -> (size(s)=w1426:i32)
                n1740 = for {
                  N: w1428 -> [_]
                  tunnel: w1431 -> [w1455]
                  tunnel: [w1453] -> w1432 mode=indexing
                  tunnel: w1428 -> [w1447]
                  i -> [w1448]
                  n1741 = Decrement(x=w1447) -> (x-1=w1445:i32)
                  n1742 = Index Array(array=w1455, index=w1448) -> (element=w1449:u8)
                  n1743 = Equal?(x=w1448, y=w1445) -> (x = y?=w1446:bool)
                  n1744 = Number To Decimal String(number=w1449) -> (decimal integer string=w1454:string)  [unwired: 1 in]
                  n1745 = Select(t="", s=w1446, f="\r") -> (s? t:f=w1451:string)
                  n1746 = Concatenate Strings(w1454, w1451) -> (w1453:string)
                }
                n1747 = for {
                  N: w1426 -> [_]
                  tunnel: w1424 -> [w1443]
                  tunnel: [w1441] -> w1425 mode=indexing
                  tunnel: w1426 -> [w1438]
                  i -> [w1439]
                  n1748 = Decrement(x=w1438) -> (x-1=w1437:i32)
                  n1749 = Index Array(array=w1443, index=w1439) -> (element=w1442:u8)
                  n1750 = Equal?(x=w1439, y=w1437) -> (x = y?=w1436:bool)
                  n1751 = Number To Decimal String(number=w1442) -> (decimal integer string=w1440:string)  [unwired: 1 in]
                  n1752 = Select(t="", s=w1436, f="\r") -> (s? t:f=w1433:string)
                  n1753 = Concatenate Strings(w1440, w1433) -> (w1441:string)
                }
                n1754 = local read "string"() -> (w1430:string)
                n1755 = Concatenate Strings(w1432) -> (w1420:string)
                n1756 = Concatenate Strings(w1425) -> (w1419:string)
                n1757 = Concatenate Strings(w1430) -> (w1427:string)
                n1758 = Equal?(x=w1420, y=w1419) -> (x = y?=w1418:bool)
                n1759 = Equal?(x=w1420, y=w1427) -> (x = y?=w1422:bool)
                n1760 = Or(x=w1422, y=w1418) -> (x .or. y?=w1421:bool)
                n1761 = case shown="True" w1421 {
                  frame False {
                  }
                  frame True {
                    n1762 = property on="ENTER THE NEW PASSWORD" class="Str"("Visible"=TRUE) -> ()  [unwired: 2 in, 2 out]
                  }
                }
              }
            }
          }
          frame #2 {
            n1763 = String To Byte Array(string="ENTER THE NEW PASSWORD") -> (unsigned byte array=w1458:u8[])
            n1764 = Search 1D Array(1D array=w1458, element=u8 10) -> (index of element=w1462:i32)  [unwired: 1 in]
            n1765 = Index Array(array=w1458, index=w1462) -> (element=w1460:u8)
            n1766 = Equal?(x=w1460, y=10) -> (x = y?=w1457:bool)
            n1767 = case shown="True" w1457 {
              frame False {
              }
              frame True {
                n1768 = local read "ENTER THE NEW PASSWORD"() -> (w1465:string)
                n1769 = String To Byte Array(string=w1465) -> (unsigned byte array=w1470:u8[])
                n1770 = Array Size(array=w1470) -> (size(s)=w1467:i32)
                n1771 = for {
                  N: w1467 -> [_]
                  tunnel: w1470 -> [w1483]
                  tunnel: [w1480] -> w1472 mode=indexing
                  tunnel: w1467 -> [w1475]
                  i -> [w1473]
                  n1772 = Index Array(array=w1483, index=w1473) -> (element=w1482:u8)
                  n1773 = Decrement(x=w1475) -> (x-1=w1476:i32)
                  n1774 = Equal?(x=w1473, y=w1476) -> (x = y?=w1477:bool)
                  n1775 = Number To Decimal String(number=w1482) -> (decimal integer string=w1481:string)  [unwired: 1 in]
                  n1776 = Select(t="", s=w1477, f="\r") -> (s? t:f=w1474:string)
                  n1777 = Concatenate Strings(w1481, w1474) -> (w1480:string)
                }
                n1778 = local write "SrvM CP"(FALSE) -> ()
                n1779 = local write "EDIT"(FALSE) -> ()
                n1780 = local read "file path"() -> (w1464:path)
                n1781 = Concatenate Strings(w1472) -> (w1466:string)
                n1782 = Delete(path (use dialog)=w1464) -> (deleted path=w1468:path)  [unwired: 4 in, 2 out]
                n1783 = call <vilib>:"Write Characters To File.vi"("append to file? (new file:F)"=FALSE, "character string"=w1466, "file path (dialog if empty)"=w1468) -> ()  [unwired: 2 in, 1 out]
              }
            }
          }
          frame #3 {
            n1784 = case shown="True" "SrvM CP" {
              frame False {
                w1486 = ""
                n1785 = property on="ENTER CURRENT PASSWORD" class="Str"("Visible"=FALSE) -> ()  [unwired: 2 in, 2 out]
                n1786 = local write "ENTER CURRENT PASSWORD"(w1486) -> ()
                n1787 = local write "ENTER THE NEW PASSWORD"(w1486) -> ()
              }
              frame True {
                n1788 = property on="ENTER THE NEW PASSWORD" class="Str"() -> ("Visible"=w1487:bool)  [unwired: 2 in, 2 out]
                n1789 = Not(x=w1487) -> (.not. x?=w1488:bool)
                n1790 = property on="ENTER CURRENT PASSWORD" class="Str"("Visible"=w1488) -> ()  [unwired: 2 in, 2 out]
              }
            }
          }
          frame #4 {
            n1791 = String To Byte Array(string="Password") -> (unsigned byte array=w1495:u8[])
            n1792 = Search 1D Array(1D array=w1495, element=u8 10) -> (index of element=w1493:i32)  [unwired: 1 in]
            n1793 = Index Array(array=w1495, index=w1493) -> (element=w1494:u8)
            n1794 = Equal?(x=w1494, y=10) -> (x = y?=w1490:bool)
            n1795 = case shown="False" w1490 {
              frame False {
              }
              frame True {
                # "password"
                # "password"
                n1796 = local read "Password"() -> (w1508:string)
                n1797 = String To Byte Array(string=w1508) -> (unsigned byte array=w1511:u8[])
                n1798 = Array Size(array=w1511) -> (size(s)=w1506:i32)
                n1799 = local read "file path"() -> (w1496:path)
                n1800 = for {
                  N: w1506 -> [_]
                  tunnel: w1511 -> [w1528]
                  tunnel: [w1526] -> w1512 mode=indexing
                  tunnel: w1506 -> [w1523]
                  i -> [w1524]
                  n1801 = Decrement(x=w1523) -> (x-1=w1522:i32)
                  n1802 = Index Array(array=w1528, index=w1524) -> (element=w1527:u8)
                  n1803 = Equal?(x=w1524, y=w1522) -> (x = y?=w1521:bool)
                  n1804 = Number To Decimal String(number=w1527) -> (decimal integer string=w1525:string)  [unwired: 1 in]
                  n1805 = Select(t="", s=w1521, f="\r") -> (s? t:f=w1518:string)
                  n1806 = Concatenate Strings(w1525, w1518) -> (w1526:string)
                }
                n1807 = String To Byte Array(string="@143$\n") -> (unsigned byte array=w1497:u8[])
                n1808 = Array Size(array=w1497) -> (size(s)=w1502:i32)
                n1809 = call <vilib>:"Read Characters From File.vi"("file path (dialog if empty)"=w1496) -> ("character string"=w1510:string)  [unwired: 5 in, 3 out]
                "string" <- w1510
                n1810 = for {
                  N: w1502 -> [_]
                  tunnel: w1497 -> [w1539]
                  tunnel: [w1537] -> w1500 mode=indexing
                  tunnel: w1502 -> [w1534]
                  i -> [w1535]
                  n1811 = Decrement(x=w1534) -> (x-1=w1533:i32)
                  n1812 = Index Array(array=w1539, index=w1535) -> (element=w1538:u8)
                  n1813 = Equal?(x=w1535, y=w1533) -> (x = y?=w1532:bool)
                  n1814 = Number To Decimal String(number=w1538) -> (decimal integer string=w1536:string)  [unwired: 1 in]
                  n1815 = Select(t="", s=w1532, f="\r") -> (s? t:f=w1529:string)
                  n1816 = Concatenate Strings(w1536, w1529) -> (w1537:string)
                }
                n1817 = Concatenate Strings(w1512) -> (w1504:string)
                n1818 = Concatenate Strings(w1510) -> (w1509:string)
                n1819 = Equal?(x=w1504, y=w1509) -> (x = y?=w1499:bool)
                n1820 = Concatenate Strings(w1500) -> (w1501:string)
                n1821 = Equal?(x=w1504, y=w1501) -> (x = y?=w1505:bool)
                n1822 = Or(x=w1499, y=w1505) -> (x .or. y?=w1498:bool)
                "x = y?" <- w1498
                n1823 = case shown="True" w1498 {
                  selector: w1498 -> [w1515 _]
                  tunnel: w1507 -> [_ _]
                  frame False {
                    n1824 = And(x=w1515, y=TRUE ("Visible")) -> (x .and. y?=w1516:bool)
                    n1825 = property on="message" class="Str"("Visible"=w1516) -> ()  [unwired: 2 in, 2 out]
                  }
                  frame True {
                    n1826 = property on="message" class="Str"("Visible"=FALSE) -> ()  [unwired: 2 in, 2 out]
                  }
                }
                n1827 = flat-sequence {
                  tunnel: [w1513] -> w1507
                  frame #0 {
                    w1513 = ""
                    n1828 = local write "Password"(w1513) -> ()
                  }
                }
              }
            }
          }
        }
        n1829 = case shown="True" "SrvM CP 2" {
          frame False {
          }
          frame True {
            n1830 = local read "FRIC. FORCE : 2"() -> (w1401:dbl)
            n1831 = local read "STROKE GAIN : 2"() -> (w1400:dbl)
            n1832 = local read "TEMPERATURE : 2"() -> (w1398:dbl)
            n1833 = local read "HUMIDITY: 2"() -> (w1396:dbl)
            n1834 = local read "DISPLACEMENT : 4"() -> (w1399:dbl)
            n1835 = local read "AIR TEMPERATURE : 2"() -> (w1397:dbl)
            n1836 = local read "TEMP INTERCEPT: 2"() -> (w1395:dbl)
            n1837 = local read "AIR TEMP INTERCEPT: 2"() -> (w1394:dbl)
            n1838 = local write "FRIC. FORCE :"(w1401) -> ()
            n1839 = local write "STROKE GAIN :"(w1400) -> ()
            n1840 = local write "TEMPERATURE :"(w1398) -> ()
            n1841 = local write "AIR TEMPERATURE :"(w1397) -> ()
            n1842 = local write "HUMIDITY:"(w1396) -> ()
            n1843 = local write "DISPLACEMENT :"(w1399) -> ()
            n1844 = local write "AIR TEMP INTERCEPT:"(w1395) -> ()
            n1845 = local write "TEMP INTERCEPT:"(w1394) -> ()
            n1846 = local write "SrvM CP 2"(FALSE ("SrvM CP 2")) -> ()
          }
        }
        n1847 = local read "STROKE GAIN : 2"() -> (w1370:dbl)
        n1848 = local read "FRIC. FORCE : 2"() -> (w1373:dbl)
        n1849 = local read "AIR TEMPERATURE : 2"() -> (w1361:dbl)
        n1850 = local read "DISPLACEMENT : 4"() -> (w1366:dbl)
        n1851 = local read "TEMPERATURE : 2"() -> (w1364:dbl)
        n1852 = local read "STROKE GAIN :"() -> (w1369:dbl)
        n1853 = local read "HUMIDITY: 2"() -> (w1357:dbl)
        n1854 = local read "FRIC. FORCE :"() -> (w1372:dbl)
        n1855 = local read "AIR TEMPERATURE :"() -> (w1360:dbl)
        n1856 = local read "DISPLACEMENT :"() -> (w1365:dbl)
        n1857 = local read "TEMPERATURE :"() -> (w1362:dbl)
        n1858 = local read "HUMIDITY:"() -> (w1356:dbl)
        n1859 = Subtract(x=w1357, y=w1356) -> (x-y=w1358:dbl)
        n1860 = Subtract(x=w1370, y=w1369) -> (x-y=w1368:dbl)
        n1861 = Subtract(x=w1373, y=w1372) -> (x-y=w1371:dbl)
        n1862 = Subtract(x=w1364, y=w1362) -> (x-y=w1363:dbl)
        n1863 = Subtract(x=w1366, y=w1365) -> (x-y=w1367:dbl)
        n1864 = Subtract(x=w1361, y=w1360) -> (x-y=w1359:dbl)
        n1865 = Divide(x=w1368, y=w1369) -> (x/y=w1388:dbl)
        n1866 = Divide(x=w1359, y=w1360) -> (x/y=w1383:dbl)
        n1867 = Divide(x=w1371, y=w1372) -> (x/y=w1391:dbl)
        n1868 = Divide(x=w1358, y=w1356) -> (x/y=w1380:dbl)
        n1869 = Divide(x=w1363, y=w1362) -> (x/y=w1384:dbl)
        n1870 = Divide(x=w1367, y=w1365) -> (x/y=w1387:dbl)
        n1871 = Multiply(x=w1388, y=100.0) -> (x*y=→"STROKE Calibration Error":dbl)
        n1872 = Multiply(x=w1383, y=100.0) -> (x*y=→"AIR TEMPERATURE  Calibration Error":dbl)
        n1873 = Multiply(x=w1391, y=100.0) -> (x*y=→"FRIC. FORCE Calibration Error":dbl)
        n1874 = Multiply(x=w1387, y=100.0) -> (x*y=→"DISPLACEMENT  Calibration Error":dbl)
        n1875 = Multiply(x=w1380, y=100.0) -> (x*y=→"HUMIDITY  Calibration Error":dbl)
        n1876 = Multiply(x=w1384, y=100.0) -> (x*y=→"TEMPERATURE  Calibration Error":dbl)
      }
    }
  }
  n1877 = while {
    tunnel: [w2841] -> _
    tunnel: [w2840] -> w49
    tunnel: w23 -> [_]
    i -> [w2841]
    stop <- w2840 stop-if-true
    n1878 = local read "Main Tab"() -> (w2826:T1)
    n1879 = local read "EDIT"() -> (w2847:bool)
    n1880 = case shown="True" w2847 {
      tunnel: [FALSE TRUE] -> w2832
      frame False {
      }
      frame True {
      }
    }
    n1881 = local read "Rate"() -> (w2846:dbl)
    n1882 = Divide(x=1.0, y=w2846) -> (x/y=w2842:dbl)
    "Time 2" <- w2842
    n1883 = property on="Time slide" class="Slide (strict)"("Scale.Range:Maximum"=2500.0) -> ()  [unwired: 2 in, 2 out]
    n1884 = local read "conststatus"() -> (w2828:dbl)
    n1885 = Equal?(x=w2826, y=T12."About" ("Main Tab")) -> (x = y?=w2838:bool)
    n1886 = property on="FF Calibration g" class="WFGraph (strict)"("Visible"=w2832) -> ()  [unwired: 2 in, 2 out]
    n1887 = property on="Lift" class="Bool (strict)"("Visible"=w2832) -> ()  [unwired: 2 in, 2 out]
    n1888 = property on="Threshold" class="DigNum (strict)"("Visible"=w2832) -> ()  [unwired: 2 in, 2 out]
    n1889 = property on="Time slide" class="Slide (strict)"("Visible"=w2832) -> ()  [unwired: 2 in, 2 out]
    n1890 = Select(t=u32 2500 ("milliseconds to wait"), s=w2838, f=u32 500 ("milliseconds to wait")) -> (s? t:f=w2836:u32)
    n1891 = Multiply(x=w2842, y=w2836) -> (x*y=w2844:dbl)
    n1892 = Wait (ms)(milliseconds to wait=u32 50) -> ()  [unwired: 1 out]
    n1893 = call "Elapsed Time2"("Time Target (s)"=w2844, "Auto Reset"=TRUE) -> ("Time has Elapsed"=w2833:bool)  [unwired: 10 in, 7 out]
    n1894 = Equal?(x=w2828, y=0.0) -> (x = y?=w2829:bool)
    n1895 = case shown="True" w2829 {
      frame False {
      }
      frame True {
        # "C:\\WinDucom\\calibrate WO 2391.dcf"
        n1896 = local write "Lan flag"(22) -> ()
        n1897 = local write "conststatus"(10.0 ("rpm value : 2")) -> ()
        n1898 = String To Path(string="C:\\LAB-IQ-NXT\\calibrate WO 2464.dcf") -> (path=w2853:path)
        n1899 = Open/Create/Replace File "Open File"(file path (use dialog)=w2853) -> (refnum out=w2851:refnum<file>)  [unwired: 5 in, 2 out]
        n1900 = for {
          N: 22 -> [_]
          tunnel: w2851 -> [w2862]
          i -> [w2856]
          (unwired) TRUE ("line mode (F)")
          n1901 = Read from Text File "Read File"(file (use dialog)=w2862) -> (text=w2861:string)  [unwired: 3 in, 3 out]
          n1902 = Match Pattern(string=w2861, regular expression="]") -> (after substring=w2859:string)  [unwired: 1 in, 3 out]
          n1903 = String Subset(string=w2861, offset (0)=5, length (rest)=10 ("length (rest)")) -> (substring=w2854:string)
          n1904 = Fract/Exp String To Number(string=w2854) -> (number=w2855:dbl)  [unwired: 3 in, 1 out]
          n1905 = Match Pattern(string=w2859, regular expression="-") -> (before substring=w2857:string)  [unwired: 1 in, 3 out]
          n1906 = case shown="2" w2856 {
            tunnel: w2855 -> [w2865 w2866 w2867 w2868 _ _ _ w2873 w2874 w2875 w2878 w2879 w2880 w2881 w2882 w2883 w2884 w2887 w2888 _ _ w2891 _]
            tunnel: w2857 -> [_ _ _ _ w2869 w2870 w2871 _ _ _ _ _ _ _ _ _ _ _ _ w2889 w2890 _ _]
            frame 0 {
              n1907 = local write "FRIC. FORCE :"(w2865) -> ()
            }
            frame 1 {
              n1908 = local write "TEMPERATURE :"(w2866) -> ()
            }
            frame 2 {
              n1909 = local write "HUMIDITY:"(w2867) -> ()
            }
            frame 3 {
              n1910 = local write "AIR TEMPERATURE :"(w2868) -> ()
            }
            frame 4 {
              n1911 = local write "Com Port 1"(w2869) -> ()
            }
            frame 5 {
              n1912 = local write "visa due"(w2870) -> ()
              n1913 = local write "Com Port 2"(w2870) -> ()
            }
            frame 6 {
              n1914 = String To Path(string=w2871) -> (path=w2872:path)
              n1915 = local write "File Path"(w2872) -> ()
              "String" <- w2871
            }
            frame 7 {
              n1916 = local write "DISPLACEMENT :"(w2873) -> ()
            }
            frame 8 {
              n1917 = local write "STROKE GAIN :"(w2874) -> ()
            }
            frame 9 {
              n1918 = local read "Stroke PID Gains"() -> (w2877:T5)
              n1919 = Bundle By Name(cluster=w2877, "Proportional Gain (Kc)"=w2875) -> (w2876:T5)
              n1920 = local write "Stroke PID Gains"(w2876) -> ()
            }
            frame 10 {
              n1921 = local write "Language Selection"(w2878) -> ()
            }
            frame 11 {
